vi "Dbin9225-7_FPGA.vi"(1 "dBin<0":bool, 2 "b":fxp<+,36,0>, 3 "a":fxp<+,36,0>) -> (0 "dBin [-0.5,0.5)":fxp<+/-,36,0>)   [LabVIEW 2021]
uses:
  <vilib>/rvi/FXPMathLib/FxpInterpret/XNode/nifxpmath_Interpret.xnode
  <vilib>/rvi/FXPMathLib/FxpSub/XNode/nifxpmath_Sub.xnode
  <vilib>/rvi/FXPMathLib/FxpAdd/XNode/nifxpmath_Add.xnode
  <vilib>/rvi/FXPMathLib/sim/FxpSim.dll
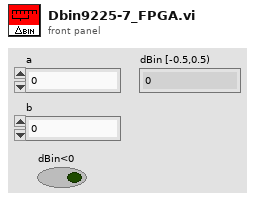
[diagram p1: front panel]
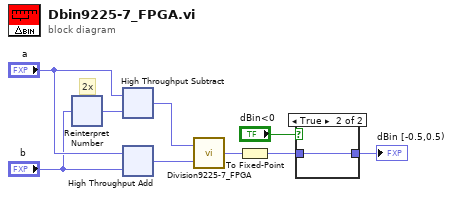
[diagram p0: block diagram]
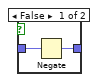
[diagram p2: hidden frame]
diagram:
  # "2x"
  n1 = xnode "Reinterpret Number"("x"="b") -> ("y"=w8:fxp<+,36,1>)
  n2 = xnode "High Throughput Subtract"("x"="a", "y"=w8) -> ("x-y"=w2:fxp<+/-,36,0>)
  n3 = xnode "High Throughput Add"("x"="a", "y"="b") -> ("x+y"=w1:fxp<+,36,1>)
  n4 = call "Division9225-7_FPGA.vi"("y <+/-49,13>"=w1, "x <+/-40,4>"=w2) -> ("x/y <+/-38,4>"=w3:fxp<+/-,48,14>)
  n5 = To Fixed-Point(number=w3) -> (fixed-point=w6:fxp<+/-,36,0>)  [unwired: 1 in]
  n6 = case shown="True" "dBin<0" {
    tunnel: [w11 w12] -> w7
    tunnel: w6 -> [w10 w12]
    frame False {
      n7 = Negate(x=w10) -> (-x=w11:fxp<+/-,36,0>)
    }
    frame True {
    }
  }
  "dBin [-0.5,0.5)" <- w7
